vi "Validate Connection.vi"(6 "validation information in":T1, 8 "error in":errorcluster, 9 "routing channel error information":T2, 10 "connection":T4, 11 "routing channel in":T3 format="%.0x") -> (0 "error out":errorcluster, 1 "veristand error out":errorcluster, 3 "routing channel out":T3 format="%.0x", 4 "validation information out":T1)   [LabVIEW 2020, in "Routing and Faulting Scripting.lvlib"]
uses:
  Routing and Faulting Scripting.lvlib
  Validation Information.ctl
  Shared/Connection.ctl
  <vilib>/NI VeriStand/Custom Device API/Custom Device Item Ref.ctl
  Routing Channel/Routing Channel Error Information.ctl
  Dependencies.llb/Routing and Faulting Shared.lvlib
  <vilib>/NI VeriStand/Custom Device API/Custom Device API.lvlib
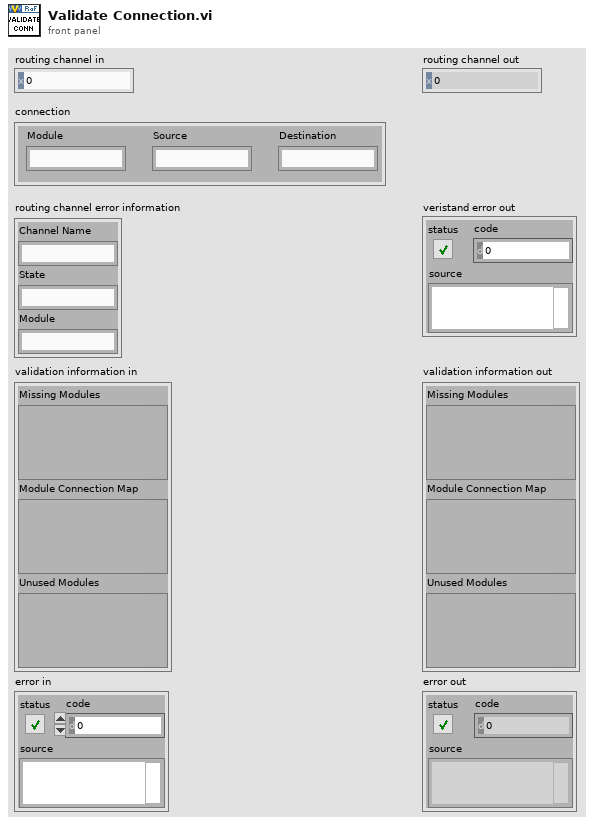
[diagram p1: front panel]
types:
  T1 = typedef "Routing and Faulting Scripting.lvlib/Validation Information.ctl" = cluster{"Missing Modules":variant, "Module Connection Map":variant, "Unused Modules":variant}
  T2 = typedef "Routing and Faulting Scripting.lvlib/Routing Channel Error Information.ctl" = cluster{"Channel Name":string, "State":string, "Module":string}
  T3 = typedef "Custom Device API.lvlib/Custom Device Item Ref.ctl" = u64
  T4 = typedef "Routing and Faulting Shared.lvlib/Connection.ctl" = cluster{"Module":string, "Source":string, "Destination":string}
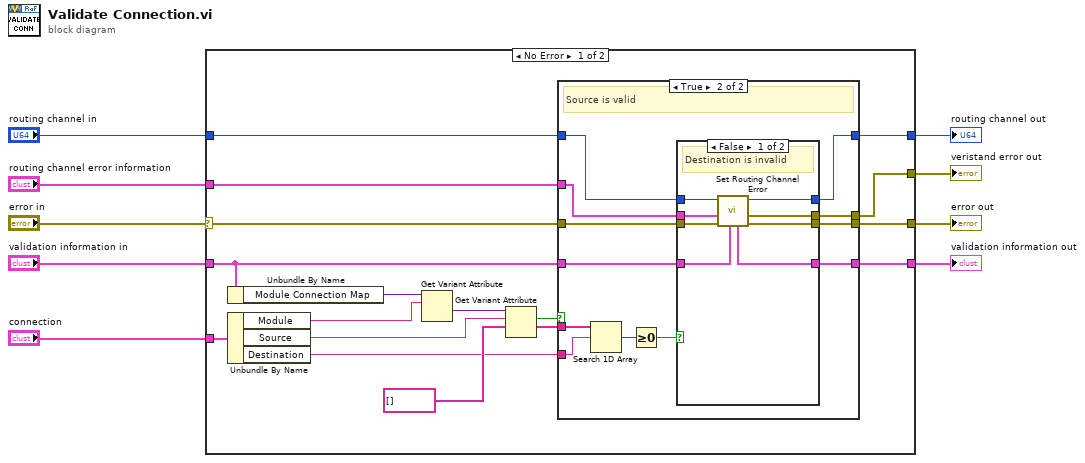
[diagram p0: block diagram]
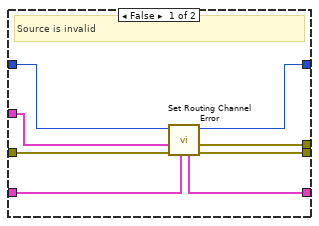
[diagram p2: hidden frame]
diagram:
  n1 = case shown="No Error" "error in" {
    selector: "error in" -> [w17 w59]
    tunnel: "validation information in" -> [w11 w58]
    tunnel: "connection" -> [w25 _]
    tunnel: "routing channel error information" -> [w16 _]
    tunnel: "routing channel in" -> [w15 w60]
    tunnel: [w14 w59] -> w4
    tunnel: [w13 w60] -> w3
    tunnel: [w12 _] -> w2
    tunnel: [w10 w58] -> w1
    frame No Error {
      n2 = Unbundle By Name(w11) -> ("Module Connection Map"=w26:variant)
      n3 = Unbundle By Name(w25) -> ("Module"=w24:string, "Source"=w22:string, "Destination"=w19:string)
      n4 = Get Variant Attribute(Variant=w26, name=w24) -> (value=w23:variant)  [unwired: 2 in, 3 out]
      n5 = Get Variant Attribute(Variant=w23, name=w22, default value (empty Variant)=string[] []) -> (found=w20:bool, value=w18:string[])  [unwired: 1 in, 2 out]
      n6 = case shown="True" w20 {
        tunnel: w19 -> [_ w45]
        tunnel: w18 -> [_ w46]
        tunnel: w17 -> [w34 w42]
        tunnel: w16 -> [w27 w41]
        tunnel: w15 -> [w32 w40]
        tunnel: [w33 w39] -> w14
        tunnel: [w31 w38] -> w13
        tunnel: [w30 w37] -> w12
        tunnel: w11 -> [w29 w36]
        tunnel: [w28 w35] -> w10
        frame False {
          # "Source is invalid"
          n7 = call "Set Routing Channel Error.vi"("validation information in"=w29, "error in"=w34, "routing channel error information"=w27, "routing channel in"=w32) -> ("error out"=w33:errorcluster, "veristand error out"=w30:errorcluster, "routing channel out"=w31:T3, "validation information out"=w28:T1)  [unwired: 4 in]
        }
        frame True {
          # "Source is valid"
          n8 = Search 1D Array(1D array=w46, element=w45) -> (index of element=w44:i32)  [unwired: 1 in]
          n9 = Greater Or Equal To 0?(x=w44) -> (x >= 0?=w43:bool)
          n10 = case shown="False" w43 {
            tunnel: w42 -> [w54 w57]
            tunnel: w41 -> [w49 _]
            tunnel: w40 -> [w53 w56]
            tunnel: [w52 w57] -> w39
            tunnel: [w51 w56] -> w38
            tunnel: [w50 _] -> w37
            tunnel: w36 -> [w48 w55]
            tunnel: [w47 w55] -> w35
            frame False {
              # "Destination is invalid"
              n11 = call "Set Routing Channel Error.vi"("validation information in"=w48, "error in"=w54, "routing channel error information"=w49, "routing channel in"=w53) -> ("error out"=w52:errorcluster, "veristand error out"=w50:errorcluster, "routing channel out"=w51:T3, "validation information out"=w47:T1)  [unwired: 4 in]
            }
            frame True {
              # "All is well"
            }
          }
        }
      }
    }
    frame Error {
    }
  }
  "error out" <- w4
  "routing channel out" <- w3
  "veristand error out" <- w2
  "validation information out" <- w1
